vi "Set_Local_Origin_Z.vi"(0 "PortNumber":u8=3) -> (1 "Received String1":string="NG\r\n", 2 "Received String2":string, 3 "OK Done":bool)   [LabVIEW 2015]
panel:
  # "Port Number 0=COM1"
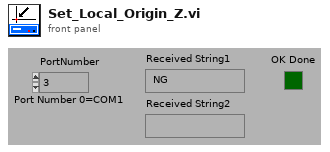
[diagram p1: front panel]
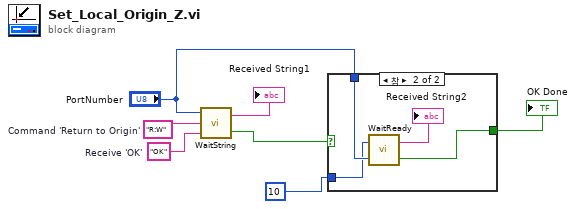
[diagram p0: block diagram]
diagram:
  w1 = "OK"  # Receive 'OK'
  w2 = "R:W"  # Command 'Return to Origin'
  n1 = call "WaitString.vi"("String to Receive"=w1, "String to Send"=w2, "PortNumber"="PortNumber") -> ("OK Done"=w4:bool, "String Received"=→"Received String1":string)
  n2 = case shown="참" w4 {
    selector: w4 -> [w8 _]
    tunnel: "PortNumber" -> [_ w12]
    tunnel: [w8 w10] -> w7
    tunnel: 10 -> [_ w9]
    frame False {
    }
    frame True {
      n3 = call "WaitReady.vi"("PortNumber"=w12, "Residence time in ms"=w9) -> ("OK Done"=w10:bool, "String Received"=→"Received String2":string)
    }
  }
  "OK Done" <- w7
